vi "Template Module Main.vi"(8 "error in":errorcluster) -> (0 "error out":errorcluster)   [LabVIEW 2018, in "Template Module.lvlib"]
doc: "This module is a free standing module of the car wash.\nIt can be stopped by the 'stop all' user event and has \na QMH architcture. The controller communicates with\nit via its named queue."
uses:
  Template Module.lvlib
  Private/ctl/Queue action--enum.ctl
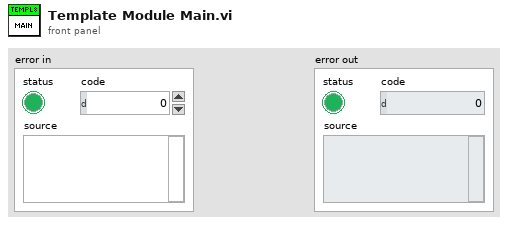
[diagram p1: front panel]
types:
  T1 = typedef "Template Module.lvlib/Queue action--enum.ctl" = enum16{"Create", "Get", "Destroy"}
  T2 = typedef "Template Module.lvlib/Message--enum.ctl" = cluster{"State":T3, "Data":variant}
  T3 = typedef "Template Module.lvlib/State--enum.ctl" = enum16{"Init", "Error", "Close"}
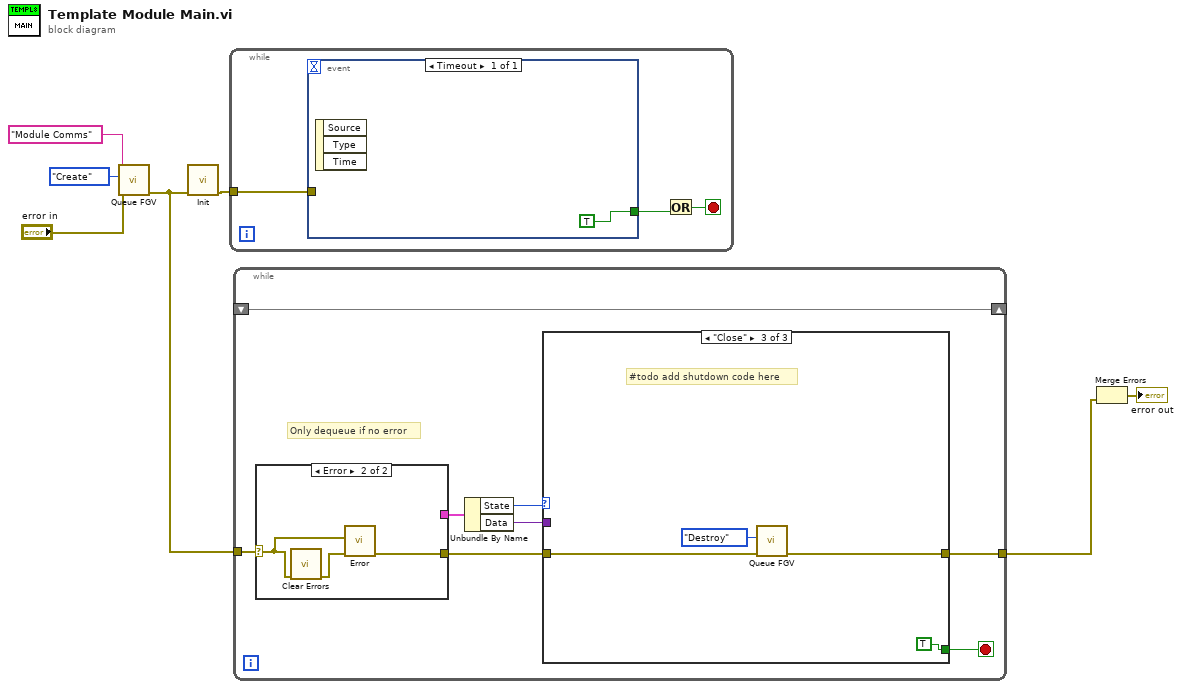
[diagram p0: block diagram]
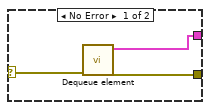
[diagram p2: hidden frame]
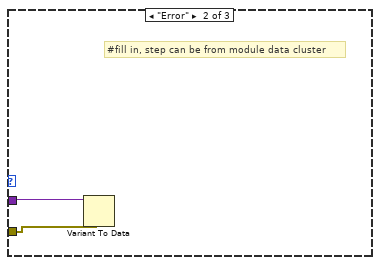
[diagram p4: hidden frame]
diagram:
  n1 = call "Queue FGV.vi"("error in"="error in", "Queue name (unnamed)"="Module Comms", "Queue Action"=Queue_action--enum."Create") -> ("error out"=w2:errorcluster)  [unwired: 7 in, 1 out]
  n2 = call "Init.vi"("error in (no error)"=w2) -> ("error out"=w3:errorcluster)  [unwired: 10 in]
  n3 = while {
    tunnel: w3 -> [w8]
    stop <- w10 stop-if-true
    n4 = event shown="[0] Timeout" {
      selector: _ -> [_]
      dyn-events: _ -> [_]
      timeout: _ -> [_]
      tunnel: [TRUE] -> w9
      tunnel: w8 -> [_]
      event Timeout {
        n5 = event-data() -> ()  [unwired: 1 in, 3 out]
      }
    }
    n6 = Or(y=w9) -> (x .or. y?=w10:bool)  [unwired: 1 in]
  }
  n7 = while {
    tunnel: [w16] -> w7
    shift-right: [w13] -> _
    shift-left: _ -> [w13]
    tunnel: w2 -> [w12]
    stop <- w15 stop-if-true
    # "Only dequeue if no error"
    n8 = case shown="Error" w12 {
      selector: w12 -> [w21 w23]
      tunnel: [w22 w25] -> w17
      tunnel: [w20 _] -> w19
      frame No Error {
        n9 = call "Dequeue element.vi"("error in (no error)"=w21) -> ("error out"=w22:errorcluster, "Message"=w20:T2)  [unwired: 9 in]
      }
      frame Error {
        n10 = call <vilib>:"Clear Errors.vi"("error in (no error)"=w23) -> ("error out"=w24:errorcluster)  [unwired: 5 in, 1 out]
        n11 = call "Error.vi"("error in (no error)"=w24, "error to pass"=w23) -> ("error out"=w25:errorcluster)  [unwired: 9 in]
      }
    }
    n12 = Unbundle By Name(w19) -> ("State"=w18:T3, "Data"=w14:variant)
    n13 = case shown="\"Close\"" w18 {
      tunnel: w17 -> [w26 w28 w31]
      tunnel: [w26 _ w30] -> w16
      tunnel: [_ _ TRUE] -> w15
      tunnel: w14 -> [_ w27 _]
      frame "Init", Default {
        # "#todo add init code here"
      }
      frame "Error" {
        # "#fill in, step can be from module data cluster"
        n14 = Variant To Data(type=w28, Variant=w27) -> ()  [unwired: 1 in, 2 out]
      }
      frame "Close" {
        # "#todo add shutdown code here"
        n15 = call "Queue FGV.vi"("error in"=w31, "Queue Action"=Queue_action--enum."Destroy") -> ("error out"=w30:errorcluster)  [unwired: 8 in, 1 out]
      }
    }
  }
  n16 = Merge Errors(w7) -> (→"error out":errorcluster)  [unwired: 1 in]
